vi "extract and prune to time range 3d.vi"(8 "error in (no error)":errorcluster, 10 "time range":dbl, 11 "queue in":refnum<queue>) -> (0 "error out":errorcluster, 2 "pruned data":T1[](array[typedef]), 3 "queue out":refnum<queue>)   [LabVIEW 2017]
uses:
  typedefs/reading3.ctl
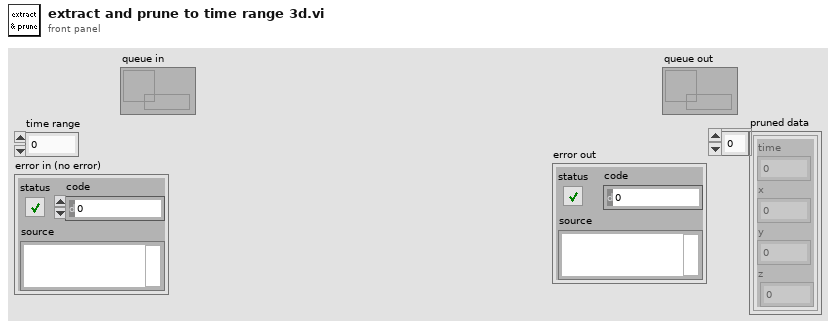
[diagram p1: front panel]
types:
  T1 = typedef "reading3.ctl" = cluster{"time":dbl, "x":dbl, "y":dbl, "z":dbl}
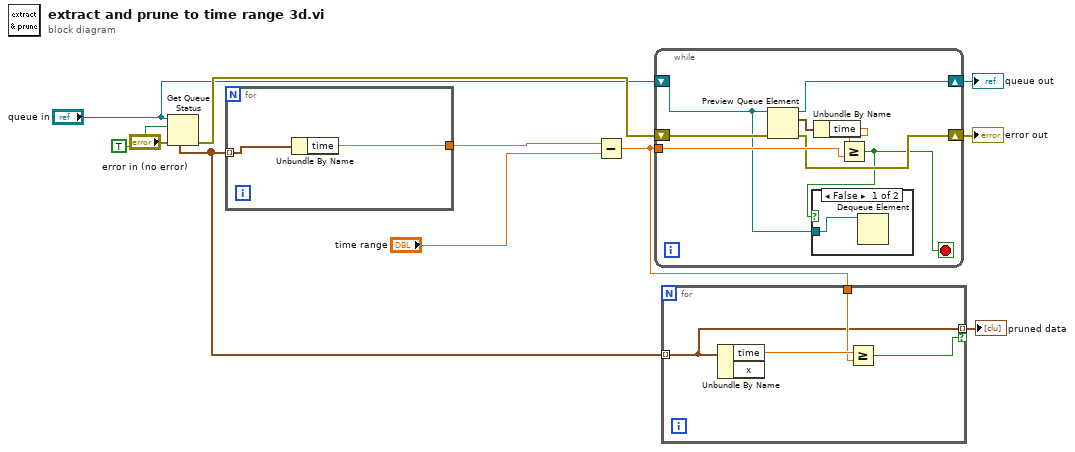
[diagram p0: block diagram]
diagram:
  n1 = Get Queue Status(queue="queue in", return elements? (F)=TRUE, error in (no error)="error in (no error)") -> (error out=w9:errorcluster, elements=w7:T1[])  [unwired: 6 out]
  n2 = for {
    tunnel: w7 -> [w13] mode=indexing
    tunnel: [w12] -> w8
    n3 = Unbundle By Name(w13) -> ("time"=w12:dbl)
  }
  n4 = Subtract(x=w8, y="time range") -> (x-y=w6:dbl)
  n5 = while {
    tunnel: w6 -> [w18]
    shift-right: [w16] -> w4
    shift-left: w9 -> [w21]
    shift-right: [w20] -> w3
    shift-left: "queue in" -> [w14]
    stop <- w15 stop-if-true
    n6 = Preview Queue Element(queue=w14, error in (no error)=w21) -> (queue out=w20:refnum<queue>, element=w17:T1, error out=w16:errorcluster)  [unwired: 1 in, 1 out]
    n7 = Unbundle By Name(w17) -> ("time"=w19:dbl)
    n8 = Greater Or Equal?(x=w19, y=w18) -> (x >= y?=w15:bool)
    n9 = case shown="False" w15 {
      tunnel: w14 -> [w22 _]
      frame False {
        n10 = Dequeue Element(queue=w22) -> ()  [unwired: 2 in, 4 out]
      }
      frame True {
      }
    }
  }
  "error out" <- w4
  "queue out" <- w3
  n11 = for {
    tunnel: w7 -> [w23] mode=indexing
    tunnel: [w23] -> w1 mode=indexing if=w24
    tunnel: w6 -> [w25]
    n12 = Unbundle By Name(w23) -> ("time"=w26:dbl)  [unwired: 1 out]
    n13 = Greater Or Equal?(x=w26, y=w25) -> (x >= y?=w24:bool)
  }
  "pruned data" <- w1
